vi "Show a status message for XX msec.vi"(8 "error in (no error)":errorcluster, 9 "Font size (24)":u32=24, 10 "Show how long (1000msecs)":u32=1000, 11 "Message":string) -> (0 "error out":errorcluster)   [LabVIEW 2013]
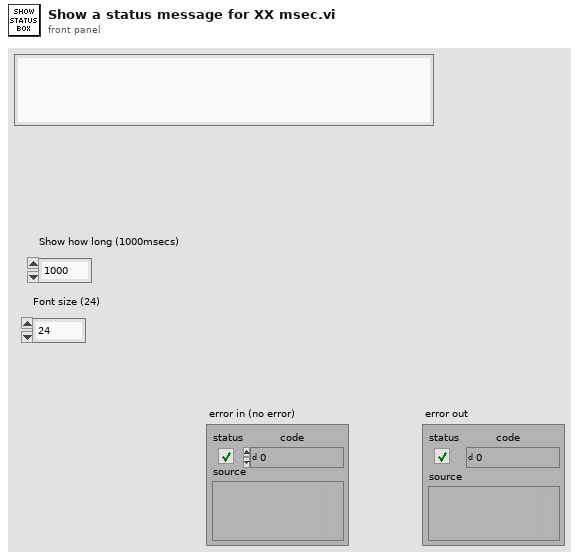
[diagram p1: front panel]
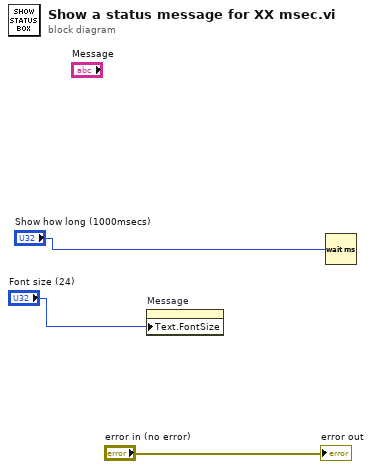
[diagram p0: block diagram]
diagram:
  n1 = property on="Message" class="Str"("Text.FontSize"="Font size (24)") -> ()  [unwired: 2 in, 2 out]
  n2 = Wait (ms)(milliseconds to wait="Show how long (1000msecs)") -> ()  [unwired: 1 out]
  "error out" <- "error in (no error)"
